vi "DAQ.Start.vi"(8 "error in":errorcluster, 10 "WFM in":waveform(dbl)[](array[waveform]), 11 "Instrument.DAQ":refnum<class "Instrument.DAQ.lvclass">) -> (0 "error out":errorcluster, 3 "Instrument.DAQ out":refnum<class "Instrument.DAQ.lvclass">)   [LabVIEW 2019, in "Instrument.Lockin.lvlib" / "Instrument.DAQ.lvclass"]
uses:
  Instrument.DAQ.lvclass
  DAQmx/typedefs/DAQmx.Commands--enum.ctl
  Instrument.DAQ.lvclass/Instrument.DAQ.ctl
  DAQmx/DAQmx.lvclass
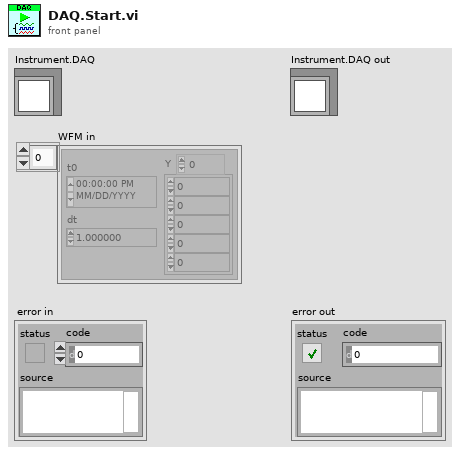
[diagram p1: front panel]
types:
  T1 = typedef "DAQmx.lvclass/DAQmx.Commands--enum.ctl" = enum16{"idle", "start", "stop", "calibrate", "auto", "exit"}
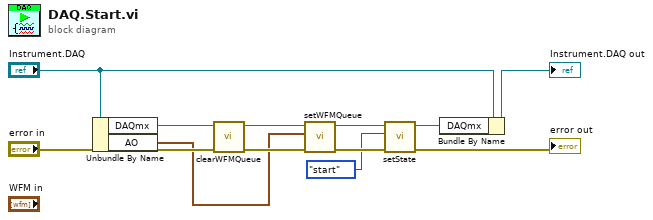
[diagram p0: block diagram]
diagram:
  n1 = Unbundle By Name("Instrument.DAQ") -> ("DAQmx"=w9:refnum<class "DAQmx.lvclass">, "AO"=w1:waveform(dbl)[])
  n2 = call "clearWFMQueue.vi"("error in (no error)"="error in", "DAQmx in"=w9) -> ("error out"=w5:errorcluster, "DAQmx out"=w8:refnum<class "DAQmx.lvclass">)  [unwired: 8 in]
  n3 = call "setWFMQueue.vi"("error in (no error)"=w5, "AO"=w1, "DAQmx in"=w8) -> ("error out"=w4:errorcluster, "DAQmx out"=w7:refnum<class "DAQmx.lvclass">)  [unwired: 7 in]
  n4 = call "setState.vi"("error in (no error)"=w4, "Command"=DAQmx.Commands--enum."start" ("State"), "DAQmx in"=w7) -> ("error out"=→"error out":errorcluster, "DAQmx out"=w12:refnum<class "DAQmx.lvclass">)  [unwired: 7 in]
  n5 = Bundle By Name(cluster="Instrument.DAQ", "DAQmx"=w12) -> (→"Instrument.DAQ out":refnum<class "Instrument.DAQ.lvclass">)
